vi "Remove Empty Folders.vi"(0 "folders path":path[](array[path]), 5 "files path":path[](array[path]), 11 "error in":errorcluster) -> (4 "required folders list":path[](array[path]), 6 "files path out":path[](array[path]), 15 "error out":errorcluster)   [LabVIEW 2021, in "Converter.lvlib"]
uses:
  Converter.lvlib
  f80cb267-0ebe-4ee9-bda0-046f5af38aa0.vi
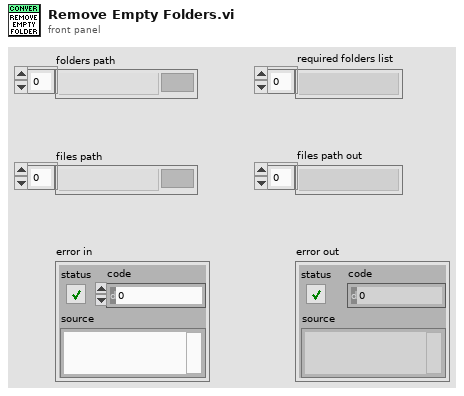
[diagram p1: front panel]
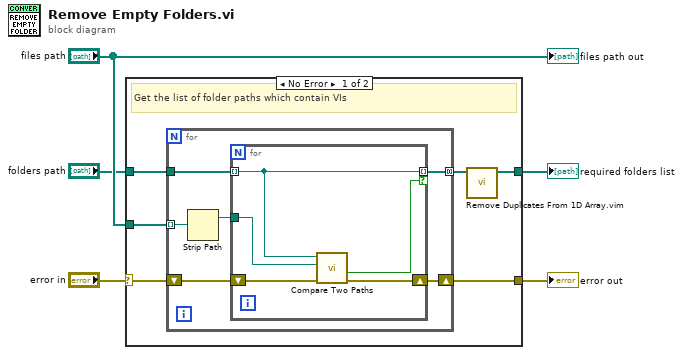
[diagram p0: block diagram]
diagram:
  n1 = case shown="No Error" "error in" {
    selector: "error in" -> [w8 w23]
    tunnel: "files path" -> [w10 _]
    tunnel: "folders path" -> [w9 _]
    tunnel: [w6 w23] -> w1
    tunnel: [w7 _] -> w2
    frame No Error {
      # "Get the list of folder paths which contain VIs"
      n2 = for {
        tunnel: w9 -> [w15]
        tunnel: w10 -> [w17] mode=indexing
        tunnel: [w14] -> w11 mode=concatenating
        shift-right: [w12] -> w6
        shift-left: w8 -> [w13]
        n3 = Strip Path(path=w17) -> (stripped path=w16:path)  [unwired: 1 out]
        n4 = for {
          tunnel: w16 -> [w22]
          tunnel: w15 -> [w21] mode=indexing
          tunnel: [w21] -> w14 mode=indexing if=w20
          shift-right: [w18] -> w12
          shift-left: w13 -> [w19]
          n5 = call <vilib>:"Compare Two Paths.vi"("error in (no error)"=w19, "Path 2"=w22, "Path 1"=w21) -> ("error out"=w18:errorcluster, "Path 2 Relative to Path 1?"=w20:bool)  [unwired: 5 in, 2 out]
        }
      }
      n6 = call "Remove Duplicates From 1D Array.vim"("array"=w11) -> ("array with duplicates removed"=w7:path[])  [unwired: 10 in]
    }
    frame Error {
      # "Pass"
    }
  }
  "error out" <- w1
  "required folders list" <- w2
  "files path out" <- "files path"
